vi "read_sample_parameters.vi"(8 "Error In":errorcluster, 10 "Sample":string, 11 "File Path":path) -> (0 "Error Out":errorcluster, 2 "Exists?":bool, 3 "Parameters":T1)   [LabVIEW 2019]
uses:
  parameters_cluster_typedef.ctl
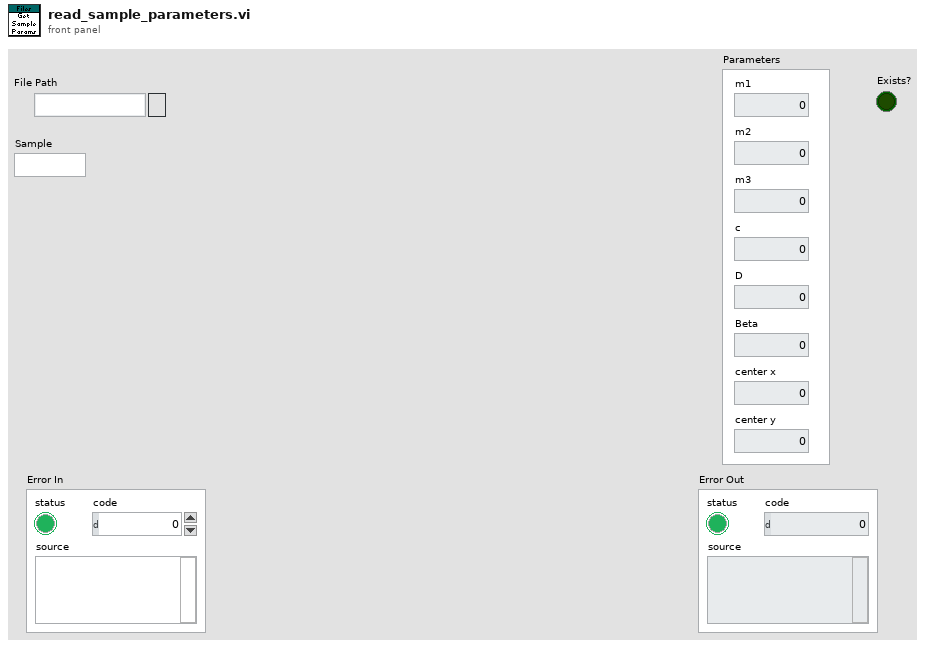
[diagram p1: front panel]
types:
  T1 = typedef "parameters_cluster_typedef.ctl" = cluster{"m1":dbl, "m2":dbl, "m3":dbl, "c":dbl, "D":dbl, "Beta":dbl, "center x":dbl, "center y":dbl}
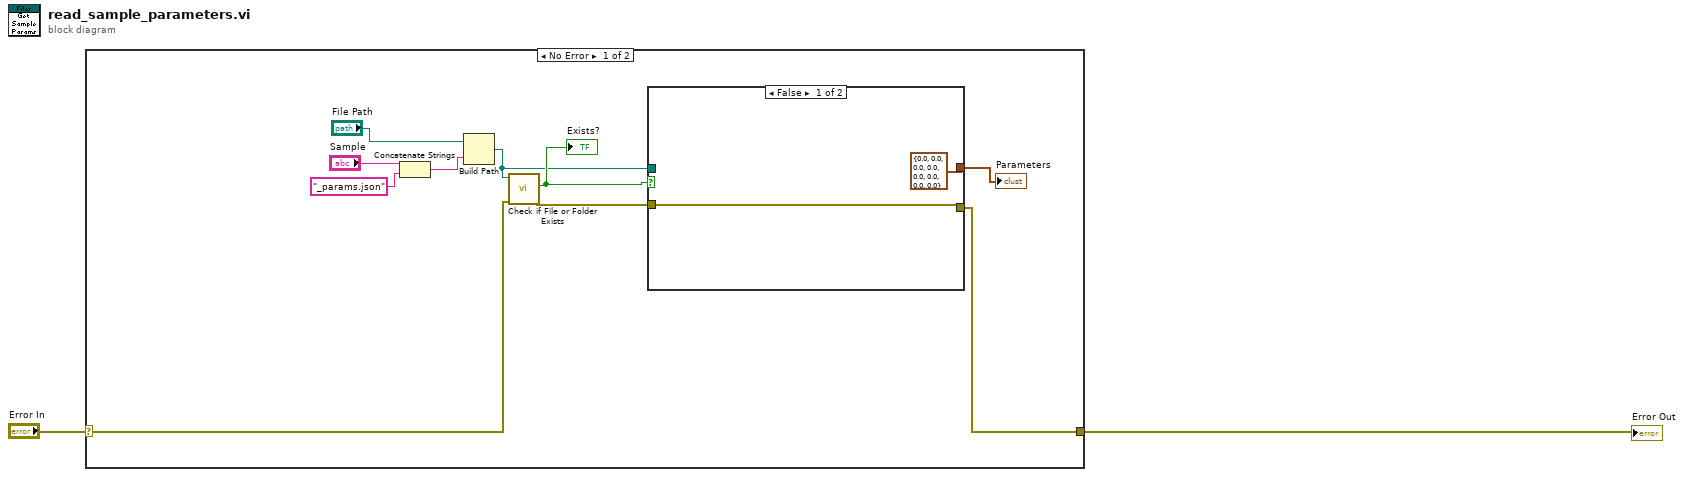
[diagram p0: block diagram]
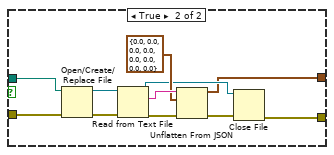
[diagram p2: hidden frame]
diagram:
  n1 = case shown="No Error" "Error In" {
    selector: "Error In" -> [w8 w26]
    tunnel: [w3 w26] -> w1
    frame No Error {
      n2 = Concatenate Strings("Sample", "_params.json" ("string")) -> (w12:string)
      n3 = Build Path(base path="File Path", name or relative path=w12) -> (appended path=w5:path)
      n4 = call <vilib>:"Check if File or Folder Exists.vi"("error in (no error)"=w8, "path"=w5) -> ("error out"=w6:errorcluster, "file or folder exists?"=w7:bool)  [unwired: 7 in, 1 out]
      "Exists?" <- w7
      n5 = case shown="False" w7 {
        tunnel: w6 -> [w14 w18]
        tunnel: w5 -> [_ w17]
        tunnel: [T1 {"m1"=0.0, "m2"=0.0, "m3"=0.0, "c"=0.0, "D"=0.0, "Beta"=0.0, "center x"=0.0, "center y"=0.0} ("Parameters") w16] -> w4
        tunnel: [w14 w15] -> w3
        frame False {
        }
        frame True {
          n6 = Open/Create/Replace File(file path (use dialog)=w17, error in=w18) -> (refnum out=w24:refnum<file>, error out=w25:errorcluster)  [unwired: 4 in, 1 out]
          n7 = Read from Text File(file (use dialog)=w24, error in=w25) -> (refnum out=w19:refnum<file>, text=w23:string, error out=w21:errorcluster)  [unwired: 2 in, 1 out]
          n8 = Unflatten From JSON(JSON string=w23, type and defaults=T1 {"m1"=0.0, "m2"=0.0, "m3"=0.0, "c"=0.0, "D"=0.0, "Beta"=0.0, "center x"=0.0, "center y"=0.0} ("Parameters"), error in (no error)=w21) -> (value=w16:T1, error out=w20:errorcluster)  [unwired: 4 in]
          n9 = Close File(refnum=w19, error in=w20) -> (error out=w15:errorcluster)  [unwired: 1 out]
        }
      }
      "Parameters" <- w4
    }
    frame Error {
    }
  }
  "Error Out" <- w1
